vi "lab4_usrp_cp_ofdm_transceiver.vi"() -> ()   [LabVIEW 2014]
uses:
  <vilib>/addons/Modulation/Digital/General/MT Generate Bits (Galois, PN Order).vi
  <vilib>/Analysis/2dsp.llb/Inverse Complex FFT.vi
  <vilib>/Analysis/2dsp.llb/Complex FFT.vi
  <vilib>/Analysis/5stat.llb/RMS (DBL).vi
  <vilib>/addons/Modulation/Digital/Support/Common/Validators/mod_Generate Bits Validate.vi
  <vilib>/addons/Modulation/Analog/support/mod_Set Error Source.vi
  var_stop.vi
  <vilib>/addons/Modulation/Digital/Support/Common/Validators/mod_Generate Filter Coefficients Validate.vi
  <vilib>/addons/Modulation/Digital/General/subVIs/mod_Generate Filter Coefficients.vi
  <vilib>/addons/Modulation/Digital/General/subVIs/mod_Generate Bits PN Sequence.vi
  <vilib>/addons/Modulation/Digital/General/MT Generate QAM System Parameters(M).vi
  <vilib>/addons/Modulation/Digital/General/MT Apply Pulse Shaping Filter (Generic).vi
  <instrlib>/niUSRP/niUSRP Write Tx Data (CDB Cluster).vi
  <vilib>/addons/Modulation/Digital/General/MT Apply Matched Filter (Generic).vi
  <vilib>/addons/Modulation/Digital/General/MT Align to Ideal Symbols (Generic).vi
  <vilib>/addons/Modulation/Digital/General/MT Map QAM Symbols to Bits.vi
  <instrlib>/niUSRP/niUSRP Fetch Rx Data (CDB Cluster).vi
  <vilib>/addons/Modulation/niDMT.lvlib
  <vilib>/Analysis/NI_AALPro.lvlib
panel:
  out "theta Graph":dbl[](graph)
  out "r Graph":dbl[](graph)
  out "Time domain ofdm signal":dbl[](graph)
  out "Frequency domain subcarrier magnitude":dbl[](graph)
  out "PAPR":dbl
  in  "M-QAM (16)":i32=16
  out "TX buffer":i32
  out "RX buffer":i32
  out "avg energy":dbl
  in  "TX on":bool=TRUE
  in  "power scale":dbl format="%#_13g"
  out "acc recieved bits":i32
  out "acc error bits":i32
  out "Packet number":u8
  out "Packet bytes":u32
  out "past 20 error bits":i32[](array[numeric])
  in  "min_len":i32=200
  in  "Threshold":dbl=-61.0 format="%#_13g"
  out "Accumulated BER":dbl
  out "found packet":bool
  in  "total bits (128)":i32=1600 caption="bits per packet"
  in  "message carriers":i32=120
  out "RX  constellation map":cdb[](graph)
  in  "pilot carrier":i32=32
  in  "cyclic length":i32=64
  in  "FFT size":i32=256
  in  "filter length (symbols)":i32=8
  in  "filter parameter":dbl=0.35 format="%.2f"
  in  "samples per symbol (16)":i32=4
  in  "pulse shaping filter (none)":T1(ring)=enum."Root Raised Cos"
  in  "stop":bool
  in  "number of samples":i64=20000
  out "coerced carrier frequency":dbl format="%#_6p"
  out "coerced IQ rate":dbl format="%#_6p"
  in  "Clocking and Synchronization:Reference Frequency Source 2":string(combo)="Internal"
  in  "Clocking and Synchronization:Reference Frequency Source":string(combo)="Internal"
  in  "RX gain":dbl format="%#_6f"
  in  "TX gain":dbl format="%#_6f"
  in  "carrier frequency":dbl=915000000.0 format="%#_6p"
  in  "IQ rate":dbl=2000000.0 format="%#_6p"
  in  "RX device names":refnum<k15>="192.168.10.3"
  in  "TX device names":refnum<k15>="192.168.10.3"
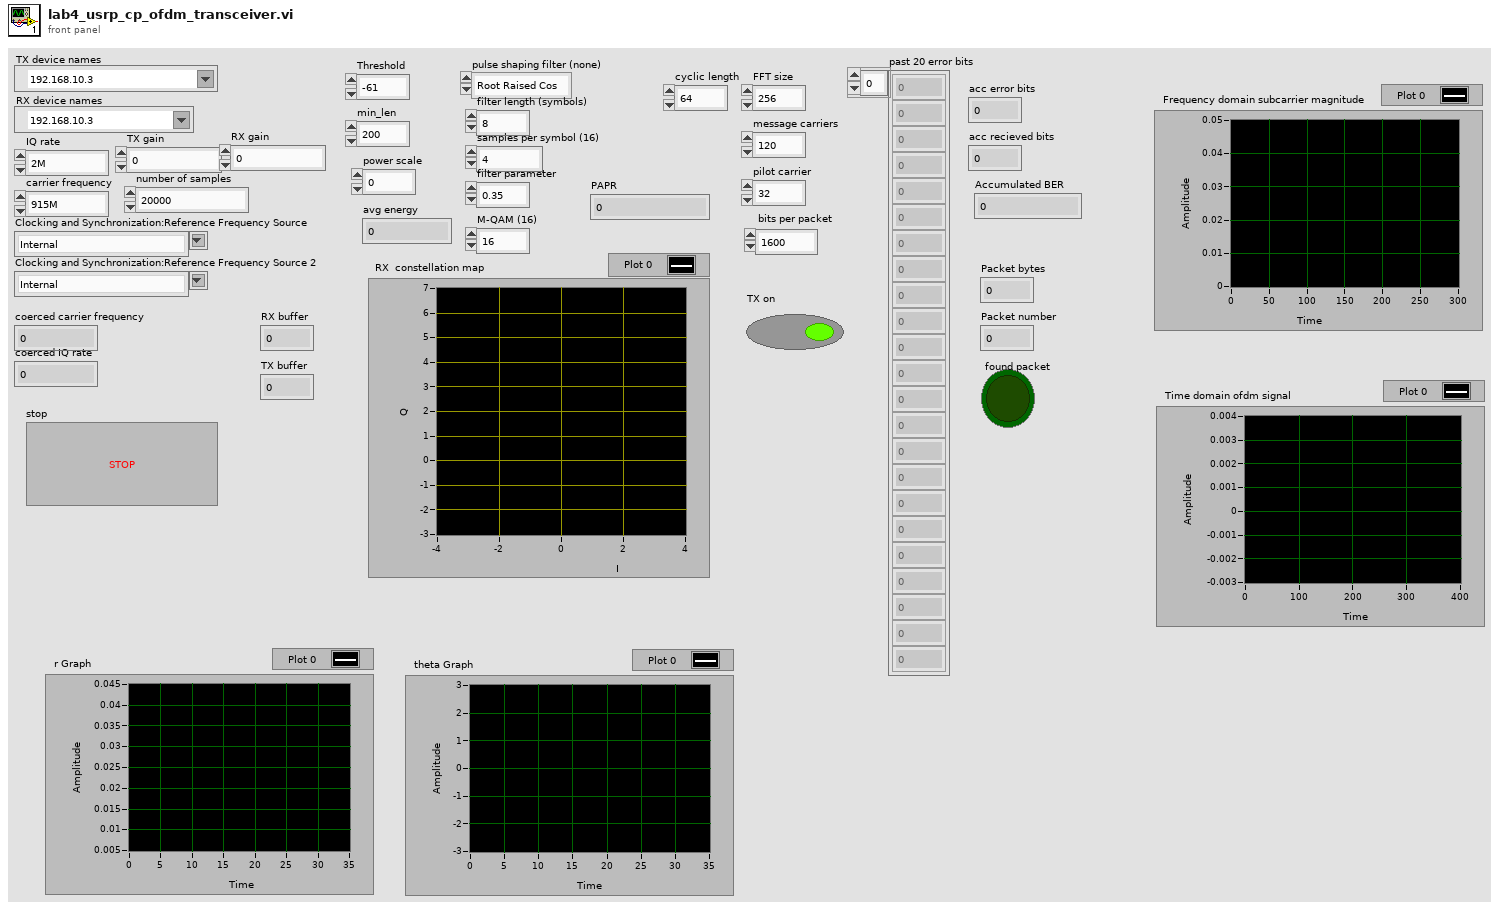
[diagram p1: front panel]
types:
  T1 = enum16{"none", "Raised Cosine", "Root Raised Cos", "Gaussian"}
  T2 = enum16{"FSK", "PSK", "QAM", "MSK", "PAM", "ASK", "CPM"}
  T3 = cluster{"samples per symbol (16)":i32, "symbol map":cdb[]}
  T4 = typedef "niAMT.lvlib/Complex Data Waveform.ctl" = cluster{"t0":dbl, "dt":dbl, "Y":cdb[]}
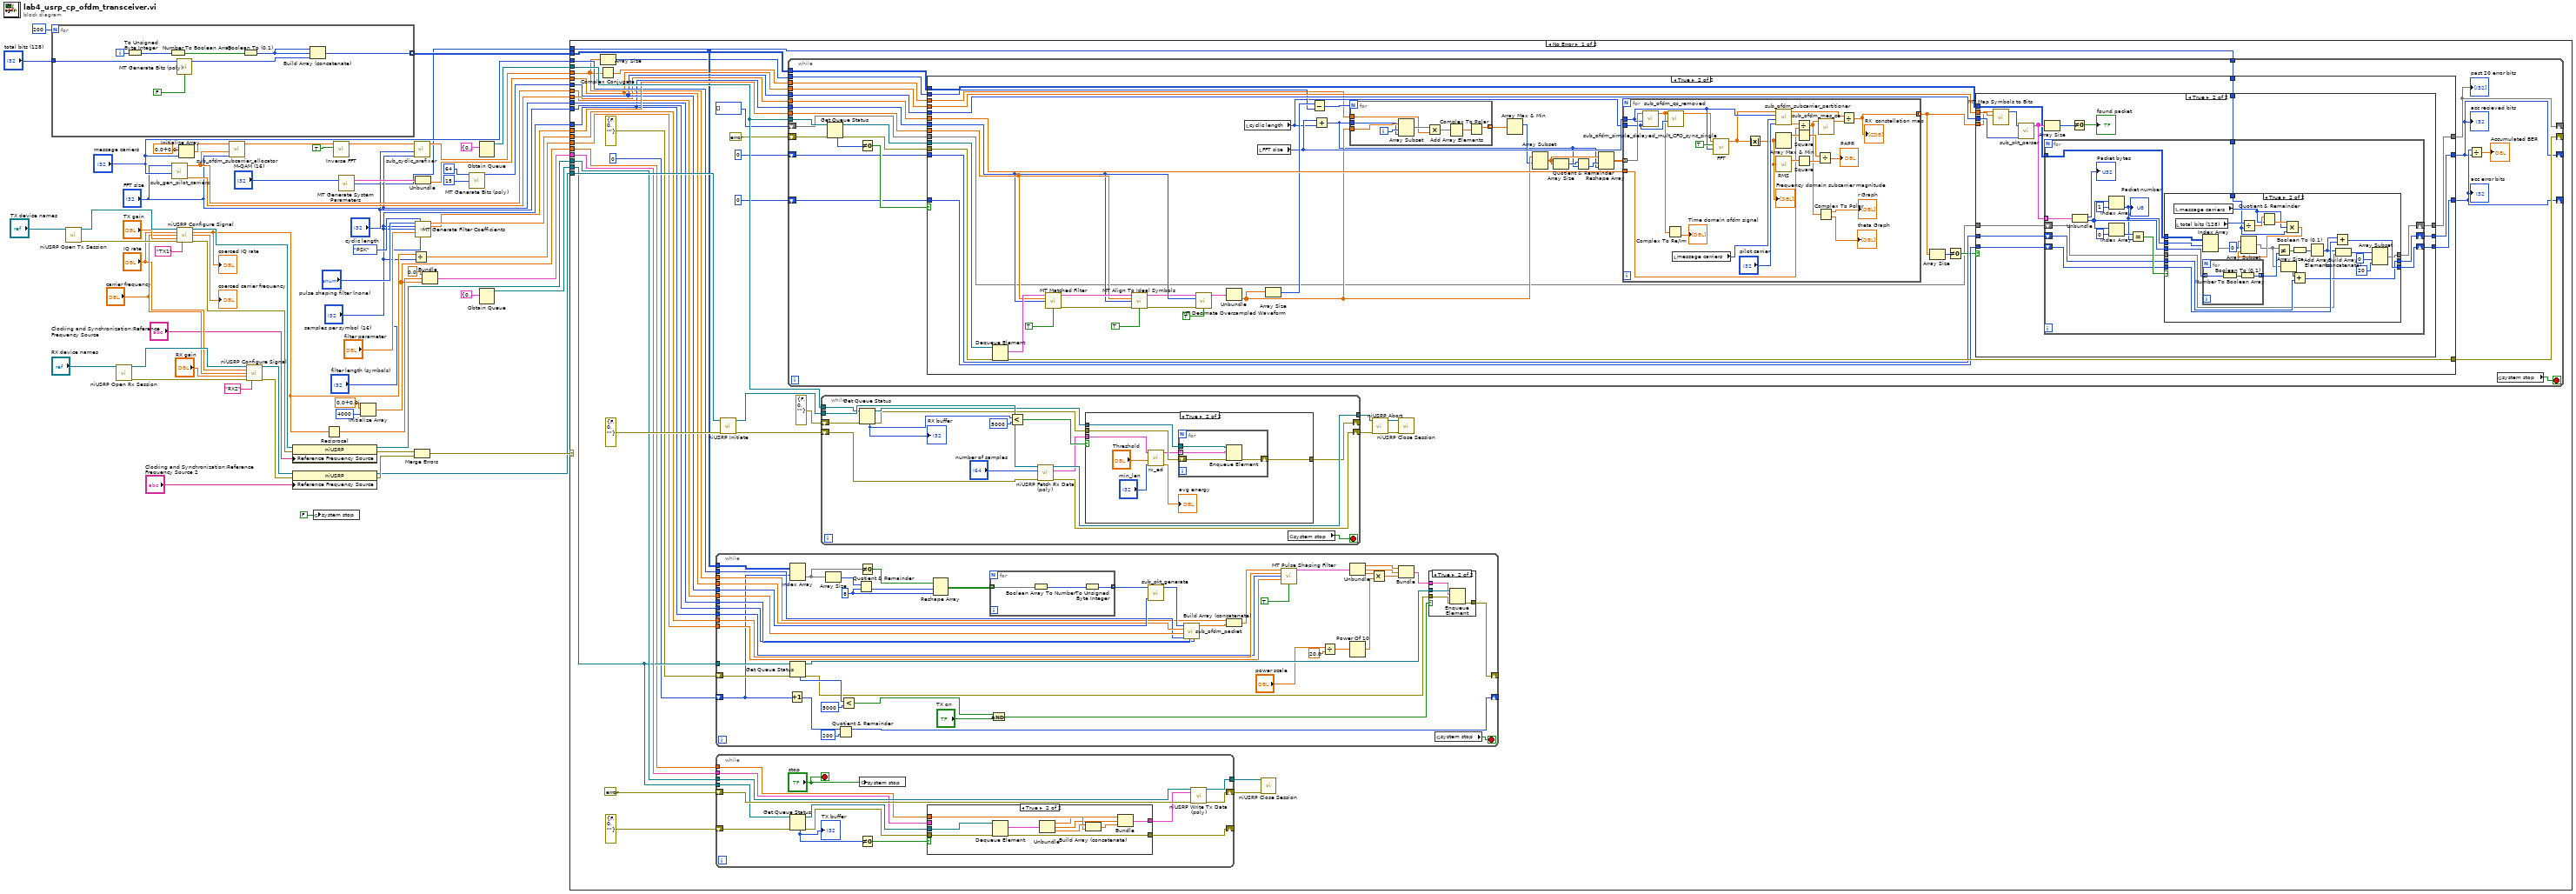
[diagram p0: block diagram]
diagram:
  n1 = for {
    N: 200 ("y") -> [_]
    tunnel: "total bits (128)" -> [w73]
    tunnel: [w66] -> w4 mode=indexing
    i -> [w71]
    n2 = To Unsigned Byte Integer(number=w71) -> (unsigned 8bit integer=w70:u8)
    n3 = Number To Boolean Array(number=w70) -> (Boolean array=w69:bool[])
    n4 = call-poly <vilib>:"MT Generate Bits (poly).vi"("total bits (128)"=w73, "reset? (T)"=FALSE) -> ("output bit stream"=w67:i8[])  [unwired: 11 in, 2 out]
    n5 = Boolean To (0,1)(Boolean=w69) -> (0, 1=w68:i16[])
    n6 = Build Array (concatenate)(w68, w68, w67) -> (w66:i16[])
  }
  n7 = call <instrlib>:"niUSRP Open Tx Session.vi"("device names"="TX device names") -> ("session handle out"=w65:refnum<k15>, "error out"=w64:errorcluster)  [unwired: 13 in]
  n8 = call <instrlib>:"niUSRP Open Rx Session.vi"("device names"="RX device names") -> ("session handle out"=w61:refnum<k15>, "error out"=w60:errorcluster)  [unwired: 13 in]
  n9 = call "sub_gen_pilot_carriers.vi"("message carrier"="message carriers", "FFT size"="FFT size") -> ("RX pilot carriers"=w17:cdb[], "TX pilot carriers"=w13:cdb[])  [unwired: 8 in]
  n10 = call <instrlib>:"niUSRP Configure Signal.vi"("session handle"=w65, "IQ rate"="IQ rate", "carrier frequency"="carrier frequency", "gain"="TX gain", "error in (no error)"=w64, "active antenna"="TX1") -> ("session handle out"=w27:refnum<k15>, "coerced IQ rate"=w16:dbl, "coerced carrier frequency"=→"coerced carrier frequency":dbl, "error out"=w26:errorcluster)  [unwired: 5 in, 1 out]
  "coerced IQ rate" <- w16
  n11 = Initialize Array(cdb 0.0+0.0i, "message carriers") -> (w19:cdb[])
  n12 = call "sub_ofdm_subcarrier_allocator.vi"("fft size"="FFT size", "pilot symbol"=w13, "message symbol"=w19) -> ("OFDM symbol"=w12:cdb[])  [unwired: 8 in]
  n13 = call <instrlib>:"niUSRP Configure Signal.vi"("session handle"=w61, "IQ rate"="IQ rate", "carrier frequency"="carrier frequency", "gain"="RX gain", "error in (no error)"=w60, "active antenna"="RX2") -> ("session handle out"=w52:refnum<k15>, "error out"=w51:errorcluster)  [unwired: 5 in, 3 out]
  n14 = property class="niUSRP"(reference=w27, error in=w26, "Reference Frequency Source"="Clocking and Synchronization:Reference Frequency Source") -> (reference out=w41:refnum<k15>, error out=w48:errorcluster)
  n15 = property class="niUSRP"(reference=w52, error in=w51, "Reference Frequency Source"="Clocking and Synchronization:Reference Frequency Source 2") -> (reference out=w43:refnum<k15>, error out=w47:errorcluster)
  n16 = global write "var_stop.vi" "system stop"(FALSE) -> ()
  n17 = Reciprocal(x=w16) -> (1/x=w36:dbl)
  n18 = call-poly <vilib>:"Inverse FFT.vi"("shift?"=TRUE, "FFT {X}"=w12) -> ("X"=w10:cdb[])  [unwired: 8 in, 1 out]
  n19 = call-poly <vilib>:"MT Generate System Parameters.vi"("M-QAM (16)"="M-QAM (16)") -> ("QAM system parameters"=w25:T3, "bits per symbol"=w1:i32)  [unwired: 12 in, 1 out]
  n20 = Initialize Array(cdb 0.0+0.0i, 4000 ("dimension size")) -> (w3:cdb[])
  n21 = Divide(x=w16, y="samples per symbol (16)") -> (x/y=w15:dbl)
  n22 = call "sub_cyclic_prefixer.vi"("FFT size"="FFT size", "CP length"="cyclic length", "time_samples"=w10) -> ("cp ofdm symbol"=w7:cdb[])  [unwired: 8 in]
  n23 = Merge Errors(w48, w47) -> (w46:errorcluster)
  n24 = Unbundle(w25) -> ("symbol map"=w24:cdb[])  [unwired: 1 out]
  n25 = call <vilib>:"MT Generate Filter Coefficients.vi"("pulse shaping filter (none)"="pulse shaping filter (none)", "modulation type"=T2."PSK", "pulse shaping samples per symbol (16)"="samples per symbol (16)", "matched samples per symbol (16)"="samples per symbol (16)", "filter parameter"="filter parameter", "filter length (symbols)"="filter length (symbols)") -> ("pulse shaping filter coefficients"=w30:dbl[], "matched filter coefficients"=w29:dbl[])  [unwired: 7 in, 1 out]
  n26 = Bundle(0.0, w36, w3) -> (w34:cluster{dbl, dbl, cdb[]})  [unwired: 1 in]
  n27 = call-poly <vilib>:"MT Generate Bits (poly).vi"("total bits (128)"=64, "PN sequence order (9)"=15) -> ("output bit stream"=w21:i8[])  [unwired: 11 in, 2 out]
  n28 = Obtain Queue(element data type=cluster{"t0":dbl, "dt":dbl, "Y":cdb[]} {"t0"=0.0, "dt"=0.0, "Y"=[]} ("data")) -> (queue out=w42:refnum<queue>)  [unwired: 4 in, 2 out]
  n29 = Obtain Queue(element data type=cluster{"t0":dbl, "dt":dbl, "Y":cdb[]} {"t0"=0.0, "dt"=0.0, "Y"=[]} ("data")) -> (queue out=w39:refnum<queue>)  [unwired: 4 in, 2 out]
  n30 = case shown="No Error" w46 {
    tunnel: w43 -> [w111 _]
    tunnel: w42 -> [w106 _]
    tunnel: w41 -> [w101 _]
    tunnel: w39 -> [w98 _]
    tunnel: w34 -> [w99 _]
    tunnel: w30 -> [w96 _]
    tunnel: w29 -> [w95 _]
    tunnel: "message carriers" -> [w92 _]
    tunnel: "FFT size" -> [w91 _]
    tunnel: w24 -> [w90 _]
    tunnel: w21 -> [w89 _]
    tunnel: w17 -> [w88 _]
    tunnel: w15 -> [w87 _]
    tunnel: "samples per symbol (16)" -> [w84 _]
    tunnel: w13 -> [w86 _]
    tunnel: "cyclic length" -> [w85 _]
    tunnel: w7 -> [w78 _]
    tunnel: w4 -> [w82 _]
    tunnel: w3 -> [w79 _]
    tunnel: w1 -> [w74 _]
    frame No Error {
      n31 = Complex Conjugate(1:w78) -> (0:w76:cdb[])
      n32 = Array Size(array=w78) -> (size(s)=w77:i32)
      n33 = while {
        tunnel: w98 -> [w153]
        shift-right: [w155] -> _
        shift-left: errorcluster {"status"=FALSE, "code"=0, "source"=""} ("error out") -> [w154]
        tunnel: w86 -> [w145]
        tunnel: w96 -> [w152]
        tunnel: w84 -> [w151]
        tunnel: w87 -> [w150]
        tunnel: w92 -> [w144]
        tunnel: w91 -> [w143]
        tunnel: w90 -> [w146]
        tunnel: w89 -> [w148]
        tunnel: w85 -> [w142]
        tunnel: w78 -> [w141]
        tunnel: w82 -> [w138]
        shift-right: [w134] -> _
        shift-left: 0 -> [w137]
        stop <- w160 stop-if-true
        w131 = 8 ("y")
        n34 = Increment(x=w137) -> (x+1=w136:i32)
        n35 = Index Array(array=w138, index (row)=w137) -> (element=w130:i16[])  [unwired: 1 in]
        n36 = Get Queue Status(queue=w153, error in (no error)=w154) -> (queue out=w157:refnum<queue>, error out=w156:errorcluster, # elements in queue=w159:i32)  [unwired: 1 in, 5 out]
        n37 = Array Size(array=w130) -> (size(s)=w133:i32)
        n38 = Quotient & Remainder(x=w136, y=200) -> (x-y*floor(x/y)=w134:i32)  [unwired: 1 out]
        n39 = Less?(x=w159, y=5000) -> (x < y?=w116:bool)
        n40 = Quotient & Remainder(x=w133, y=w131) -> (floor(x/y)=w132:i32)  [unwired: 1 out]
        n41 = Not Equal To 0?(x=w130) -> (x != 0?=w129:bool[])
        n42 = Reshape Array(w129, w132, w131) -> (w128:bool[][])
        n43 = for {
          tunnel: w128 -> [w163] mode=indexing
          tunnel: [w161] -> w127 mode=indexing
          n44 = Boolean Array To Number(Boolean array=w163) -> (number=w162:u32)
          n45 = To Unsigned Byte Integer(number=w162) -> (unsigned 8bit integer=w161:u8)
        }
        n46 = And(x=w116, y="TX on") -> (x .and. y?=w114:bool)
        n47 = call "sub_pkt_generate.vi"("accesscode (bit)"=w148, "byte stream"=w127) -> ("bit pkt"=w147:i16[])  [unwired: 9 in]
        n48 = call "sub_ofdm_packet.vi"("CP length"=w142, "FFT size"=w143, "message carriers"=w144, "pilot symbol"=w145, "symbol map"=w146, "packet"=w147) -> ("ofdm packet"=w140:cdb[])  [unwired: 5 in]
        n49 = Build Array (concatenate)(w141, w140) -> (w139:cdb[])
        n50 = call-poly <vilib>:"MT Pulse Shaping Filter.vi"("symbols"=w139, "pulse shaping filter coefficients"=w152, "samples per symbol (16)"=w151, "symbol rate (Hz)"=w150, "reset? (T)"=TRUE) -> ("output complex waveform"=w123:T4)  [unwired: 9 in, 1 out]
        n51 = Divide(x="power scale", y=20.0) -> (x/y=w124:dbl)
        n52 = Unbundle(w123) -> ("t0"=w118:dbl, "dt"=w119:dbl, "Y"=w122:cdb[])
        n53 = Power Of 10(x=w124) -> (10^x=w121:dbl)
        n54 = Multiply(x=w122, y=w121) -> (x*y=w120:cdb[])
        n55 = Bundle("t0"=w118, "dt"=w119, w120) -> (w117:cluster{"t0":dbl, "dt":dbl, cdb[]})  [unwired: 1 in]
        n56 = case shown="True" w114 {
          tunnel: w157 -> [_ w168]
          tunnel: w156 -> [w164 w167]
          tunnel: [w164 w166] -> w155
          tunnel: w117 -> [_ w165]
          frame False {
          }
          frame True {
            n57 = Enqueue Element(queue=w168, element=w165, error in (no error)=w167) -> (error out=w166:errorcluster)  [unwired: 1 in, 2 out]
          }
        }
        n58 = global read "var_stop.vi" "system stop"() -> (w160:bool)
      }
      n59 = while {
        tunnel: [w378] -> w104
        shift-right: [w377] -> w103
        shift-left: errorcluster {"status"=FALSE, "code"=0, "source"=""} ("error out") -> [w375]
        tunnel: w101 -> [w376]
        tunnel: w98 -> [w374]
        shift-right: [w368] -> _
        shift-left: errorcluster {"status"=FALSE, "code"=0, "source"=""} ("error out") -> [w373]
        tunnel: w99 -> [w367]
        tunnel: w79 -> [w366]
        stop <- "stop" stop-if-true
        n60 = Get Queue Status(queue=w374, error in (no error)=w373) -> (queue out=w370:refnum<queue>, error out=w371:errorcluster, # elements in queue=w372:i32)  [unwired: 1 in, 5 out]
        "TX buffer" <- w372
        n61 = global write "var_stop.vi" "system stop"("stop") -> ()
        n62 = Not Equal To 0?(x=w372) -> (x != 0?=w365:bool)
        n63 = case shown="True" w365 {
          tunnel: w371 -> [w381 w390]
          tunnel: w370 -> [_ w391]
          tunnel: [w380 w382] -> w369
          tunnel: [w381 w389] -> w368
          tunnel: w367 -> [w380 _]
          tunnel: w366 -> [_ w386]
          frame False {
          }
          frame True {
            n64 = Dequeue Element(queue=w391, error in (no error)=w390) -> (element=w388:cluster{"t0":dbl, "dt":dbl, "Y":cdb[]}, error out=w389:errorcluster)  [unwired: 1 in, 2 out]
            n65 = Unbundle(w388) -> ("t0"=w383:dbl, "dt"=w384:dbl, "Y"=w387:cdb[])
            n66 = Build Array (concatenate)(w387, w386) -> (w385:cdb[])
            n67 = Bundle("t0"=w383, "dt"=w384, w385) -> (w382:cluster{"t0":dbl, "dt":dbl, cdb[]})  [unwired: 1 in]
          }
        }
        n68 = call-poly <instrlib>:"niUSRP Write Tx Data (poly).vi"("session handle"=w376, "data"=w369, "error in (no error)"=w375) -> ("session handle out"=w378:refnum<k15>, "error out"=w377:errorcluster)  [unwired: 11 in]
      }
      n69 = call <instrlib>:"niUSRP Initiate.vi"("session handle"=w111, "error in (no error)"=errorcluster {"status"=FALSE, "code"=0, "source"=""}) -> ("session handle out"=w113:refnum<k15>, "error out"=w112:errorcluster)  [unwired: 12 in]
      n70 = while {
        tunnel: w106 -> [w187]
        shift-right: [w185] -> _
        shift-left: errorcluster {"status"=FALSE, "code"=0, "source"=""} ("error out") -> [w186]
        tunnel: w95 -> [w184]
        tunnel: w84 -> [w183]
        tunnel: w88 -> [w182]
        tunnel: w90 -> [w181]
        tunnel: w89 -> [w180]
        tunnel: w82 -> [w179]
        shift-right: [w175] -> _
        shift-left: 0 -> [w177]
        shift-right: [w176] -> _
        shift-left: 0 -> [w178]
        tunnel: w77 -> [w173]
        tunnel: w76 -> [w172]
        shift-right: [w170] -> _
        shift-left: i32[] [] -> [w171]
        tunnel: w74 -> [w169]
        stop <- w192 stop-if-true
        n71 = Get Queue Status(queue=w187, error in (no error)=w186) -> (queue out=w188:refnum<queue>, error out=w189:errorcluster, # elements in queue=w191:i32)  [unwired: 1 in, 5 out]
        n72 = Not Equal To 0?(x=w191) -> (x != 0?=w190:bool)
        n73 = case shown="True" w190 {
          tunnel: w189 -> [w196 w238]
          tunnel: w188 -> [_ w237]
          tunnel: [w196 w236] -> w185
          tunnel: w184 -> [_ w228]
          tunnel: w183 -> [_ w227]
          tunnel: w182 -> [_ w231]
          tunnel: w181 -> [_ w223]
          tunnel: w180 -> [_ w222]
          tunnel: w179 -> [_ w221]
          tunnel: w178 -> [w195 w220]
          tunnel: w177 -> [w194 w219]
          tunnel: [w195 w218] -> w176
          tunnel: [w194 w217] -> w175
          tunnel: w173 -> [_ w212]
          tunnel: w172 -> [_ w208]
          tunnel: w171 -> [w193 w199]
          tunnel: [w193 w198] -> w170
          tunnel: w169 -> [_ w197]
          frame False {
          }
          frame True {
            n74 = Dequeue Element(queue=w237, error in (no error)=w238) -> (element=w235:cluster{"t0":dbl, "dt":dbl, "Y":cdb[]}, error out=w236:errorcluster)  [unwired: 1 in, 2 out]
            n75 = call-poly <vilib>:"MT Matched Filter.vi"("input complex waveform"=w235, "matched filter coefficients"=w228, "samples per symbol (16)"=w227, "reset? (T)"=TRUE) -> ("output complex waveform"=w230:T4, "error out"=w229:errorcluster)  [unwired: 10 in]
            n76 = call-poly <vilib>:"MT Align To Ideal Symbols.vi"("input complex waveform"=w230, "matched filter coefficients"=w228, "samples per symbol (16)"=w227, "error in (no error)"=w229, "reset? (T)"=TRUE) -> ("output complex waveform"=w225:T4, "error out"=w224:errorcluster)  [unwired: 8 in, 1 out]
            n77 = call <vilib>:"MT Decimate Oversampled Waveform.vi"("input complex waveform"=w225, "decimation factor"=w227, "error in (no error)"=w224, "reset? (T)"=TRUE) -> ("output complex waveform"=w233:T4)  [unwired: 10 in, 1 out]
            n78 = Unbundle(w233) -> ("Y"=w206:cdb[])  [unwired: 2 out]
            n79 = local read "cyclic length"() -> (w209:i32)
            n80 = local read "FFT size"() -> (w210:i32)
            n81 = Array Size(array=w206) -> (size(s)=w213:i32)
            n82 = Subtract(x=w213, y=w212) -> (x-y=w211:i32)
            n83 = Add(x=w210, y=w209) -> (x+y=w201:i32)
            n84 = for {
              N: w211 -> [_]
              tunnel: w206 -> [w246]
              tunnel: w201 -> [w244]
              tunnel: w208 -> [w242]
              tunnel: [w239] -> w207 mode=indexing
              i -> [w245]
              n85 = Array Subset(array=w246, index=w245, length=w244) -> (w243:cdb[])
              n86 = Multiply(x=w243, y=w242) -> (x*y=w241:cdb[])
              n87 = Add Array Elements(numeric array=w241) -> (sum=w240:cdb)
              n88 = Complex To Polar(r * e^(i*theta)=w240) -> (r=w239:dbl)  [unwired: 1 out]
            }
            n89 = Array Max & Min(array=w207) -> (max index (indices)=w205:i32)  [unwired: 3 out]
            n90 = Array Subset(array=w206, index=w205) -> (w203:cdb[])  [unwired: 1 in]
            n91 = Array Size(array=w203) -> (size(s)=w204:i32)
            n92 = Quotient & Remainder(x=w204, y=w201) -> (floor(x/y)=w202:i32)  [unwired: 1 out]
            n93 = Reshape Array(w203, w202, w201) -> (w200:cdb[][])
            n94 = for {
              tunnel: w200 -> [w330] mode=indexing
              tunnel: w209 -> [w328]
              tunnel: w210 -> [w329]
              tunnel: [w333] -> w216 mode=concatenating
              tunnel: w231 -> [w314]
              n95 = call "sub_ofdm_simple_delayed_mult_CFO_sync_single.vi"("CP length"=w328, "FFT size"=w329, "time samples"=w330) -> ("sync ofdm symbol"=w318:cdb[])  [unwired: 8 in]
              n96 = call "sub_ofdm_cp_removed.vi"("CP length"=w328, "time ofdm symbol"=w318) -> ("cp removed ofdm symbol"=w320:cdb[])  [unwired: 9 in]
              n97 = Complex To Re/Im(x + iy=w318) -> (y=→"Time domain ofdm signal":dbl[])  [unwired: 1 out]
              n98 = local read "message carriers"() -> (w332:i32)
              n99 = call-poly <vilib>:"FFT.vi"("FFT size"=w329, "shift?"=TRUE, "X"=w320) -> ("FFT {X}"=w327:cdb[])  [unwired: 7 in, 1 out]
              n100 = Absolute Value(x=w327) -> (abs(x)=w321:dbl[])
              "Frequency domain subcarrier magnitude" <- w321
              n101 = call "sub_ofdm_subcarrier_partitioner.vi"("pilot carrier"="pilot carrier", "message carrier"=w332, "FFT size"=w329, "received symbol"=w327) -> ("pilot subcarriers"=w313:cdb[], "message subcarriers"=w331:cdb[])  [unwired: 6 in]
              n102 = Array Max & Min(array=w321) -> (max value=w326:dbl)  [unwired: 3 out]
              n103 = call-poly <vilib>:"RMS.vi"("X"=w321) -> ("rms value"=w324:dbl)  [unwired: 1 out]
              n104 = Divide(x=w313, y=w314) -> (x/y=w317:cdb[])
              n105 = Square(x=w326) -> (x^2=w325:dbl)
              n106 = Square(x=w324) -> (x^2=w323:dbl)
              n107 = Divide(x=w325, y=w323) -> (x/y=→"PAPR":dbl)
              n108 = call "sub_ofdm_mes_ce.vi"("ZF channel estimates"=w317) -> ("interpolated mes carrier CE"=w334:cdb[])  [unwired: 10 in]
              n109 = Complex To Polar(r * e^(i*theta)=w317) -> (r=→"r Graph":dbl[], theta=→"theta Graph":dbl[])
              n110 = Divide(x=w331, y=w334) -> (x/y=w333:cdb[])
              "RX  constellation map" <- w333
            }
            n111 = Array Size(array=w216) -> (size(s)=w215:i32)
            n112 = Not Equal To 0?(x=w215) -> (x != 0?=w214:bool)
            n113 = case shown="True" w214 {
              tunnel: w223 -> [_ w264]
              tunnel: w222 -> [_ w262]
              tunnel: w221 -> [_ w258]
              tunnel: w220 -> [w249 w257]
              tunnel: w219 -> [w248 w256]
              tunnel: [w249 w255] -> w218
              tunnel: [w248 w254] -> w217
              tunnel: w216 -> [_ w253]
              tunnel: w199 -> [w247 w252]
              tunnel: [w247 w251] -> w198
              tunnel: w197 -> [_ w250]
              frame False {
              }
              frame True {
                n114 = call-poly <vilib>:"MT Map Symbols to Bits.vi"("symbols"=w253, "symbol map"=w264) -> ("output bit stream"=w263:i8[])  [unwired: 12 in, 1 out]
                n115 = call "sub_pkt_parser.vi"("accesscode (bit)"=w262, "bitstream"=w263) -> ("parsed packet"=w259:cluster{"t":u32, "byte_array":u8[]}[])  [unwired: 9 in]
                n116 = Array Size(array=w259) -> (size(s)=w261:i32)
                n117 = for {
                  tunnel: w259 -> [w280] mode=indexing
                  tunnel: w258 -> [w274]
                  shift-right: [w271] -> w255
                  shift-left: w257 -> [w272]
                  shift-right: [w269] -> w254
                  shift-left: w256 -> [w270]
                  shift-right: [w267] -> w251
                  shift-left: w252 -> [w268]
                  tunnel: w250 -> [w265]
                  n118 = Unbundle(w280) -> ("t"=→"Packet bytes":u32, "byte_array"=w275:u8[])
                  n119 = Index Array(array=w275, index=1) -> (element=w273:u8)
                  "Packet number" <- w273
                  n120 = Index Array(array=w275, index=0) -> (element=w277:u8)
                  n121 = Equal?(x=w277, y=w273) -> (x = y?=w276:bool)
                  n122 = case shown="True" w276 {
                    tunnel: w275 -> [_ w295]
                    tunnel: w274 -> [_ w309]
                    tunnel: w273 -> [_ w308]
                    tunnel: w272 -> [w283 w305]
                    tunnel: [w283 w304] -> w271
                    tunnel: w270 -> [w282 w303]
                    tunnel: [w282 w302] -> w269
                    tunnel: w268 -> [w281 w301]
                    tunnel: [w281 w296] -> w267
                    tunnel: w265 -> [_ w290]
                    frame False {
                    }
                    frame True {
                      n123 = local read "message carriers"() -> (w291:i32)
                      n124 = local read "total bits (128)"() -> (w294:i32)
                      n125 = Index Array(array=w309, index (row)=w308) -> (element=w289:i16[])  [unwired: 1 in]
                      n126 = for {
                        tunnel: w295 -> [w312] mode=indexing
                        tunnel: [w310] -> w286 mode=concatenating
                        n127 = Number To Boolean Array(number=w312) -> (Boolean array=w311:bool[])
                        n128 = Boolean To (0,1)(Boolean=w311) -> (0, 1=w310:i16[])
                      }
                      n129 = Divide(x=w294, y=w290) -> (x/y=w293:dbl)
                      n130 = Quotient & Remainder(x=w293, y=w291) -> (floor(x/y)=w292:dbl)  [unwired: 1 out]
                      n131 = Compound Arithmetic op=MULTIPLY(w292, w291, w290) -> (w287:dbl)
                      n132 = Array Subset(array=w289, index=0, length=w287) -> (w285:i16[])
                      n133 = Not Equal?(x=w285, y=w286) -> (x != y?=w307:bool[])
                      n134 = Array Size(array=w285) -> (size(s)=w284:i32)
                      n135 = Boolean To (0,1)(Boolean=w307) -> (0, 1=w306:i16[])
                      n136 = Add(x=w284, y=w303) -> (x+y=w302:i32)
                      n137 = Add Array Elements(numeric array=w306) -> (sum=w300:i16)
                      n138 = Add(x=w300, y=w305) -> (x+y=w304:i32)
                      n139 = Build Array (concatenate)(w300, w301) -> (w299:i32[])
                      n140 = Array Subset(array=w299, index=0, length=20) -> (w296:i32[])
                    }
                  }
                }
                n141 = Not Equal To 0?(x=w261) -> (x != 0?=→"found packet":bool)
              }
            }
          }
        }
        "past 20 error bits" <- w170
        "acc error bits" <- w176
        "acc recieved bits" <- w175
        n142 = Divide(x=w176, y=w175) -> (x/y=→"Accumulated BER":dbl)
        n143 = global read "var_stop.vi" "system stop"() -> (w192:bool)
      }
      n144 = while {
        tunnel: w113 -> [w351]
        shift-right: [w344] -> w108
        shift-left: w112 -> [w350]
        tunnel: [w345] -> w109
        tunnel: w106 -> [w341]
        shift-right: [w339] -> _
        shift-left: errorcluster {"status"=FALSE, "code"=0, "source"=""} ("error out") -> [w338]
        stop <- w337 stop-if-true
        n145 = Get Queue Status(queue=w341, error in (no error)=w338) -> (queue out=w342:refnum<queue>, error out=w340:errorcluster, # elements in queue=w348:i32)  [unwired: 1 in, 5 out]
        "RX buffer" <- w348
        n146 = Less?(x=w348, y=5000) -> (x < y?=w346:bool)
        n147 = call-poly <instrlib>:"niUSRP Fetch Rx Data (poly).vi"("session handle"=w351, "number of samples"="number of samples", "error in (no error)"=w350) -> ("session handle out"=w345:refnum<k15>, "data"=w343:cluster{"t0":dbl, "dt":dbl, "Y":cdb[]}, "error out"=w344:errorcluster)  [unwired: 9 in, 1 out]
        n148 = case shown="True" w346 {
          tunnel: w343 -> [_ w357]
          tunnel: w342 -> [_ w358]
          tunnel: w340 -> [w352 w360]
          tunnel: [w352 w359] -> w339
          frame False {
          }
          frame True {
            n149 = call "rx_ed.vi"("min_len"="min_len", "Threshold"="Threshold", "Wavefrom"=w357) -> ("avg energy"=→"avg energy":dbl, "extract wav"=w354:cluster{"t0":dbl, "dt":dbl, cdb[]}[])  [unwired: 7 in]
            n150 = for {
              tunnel: w358 -> [w362]
              shift-right: [w363] -> w359
              shift-left: w360 -> [w364]
              tunnel: w354 -> [w361] mode=indexing
              n151 = Enqueue Element(queue=w362, element=w361, error in (no error)=w364) -> (error out=w363:errorcluster)  [unwired: 1 in, 2 out]
            }
          }
        }
        n152 = global read "var_stop.vi" "system stop"() -> (w337:bool)
      }
      n153 = call <instrlib>:"niUSRP Close Session.vi"("session handle"=w104, "error in (no error)"=w103) -> ()  [unwired: 13 in, 1 out]
      n154 = call <instrlib>:"niUSRP Abort.vi"("session handle"=w109, "error in (no error)"=w108) -> ("session handle out"=w94:refnum<k15>, "error out"=w93:errorcluster)  [unwired: 12 in]
      n155 = call <instrlib>:"niUSRP Close Session.vi"("session handle"=w94, "error in (no error)"=w93) -> ()  [unwired: 13 in, 1 out]
    }
    frame Error {
    }
  }
